vi "Setup.Numeric.Hide.vi"(8 "error in (no error)":errorcluster, 11 "Digital in":refnum<vi>) -> (0 "error out":errorcluster)   [LabVIEW 2015, in "Workspace.Obejct.Radio.lvlib"]
uses:
  Workspace.Obejct.Radio.lvlib
  <vilib>/Utility/miscctls.llb/LVPositionTypeDef.ctl
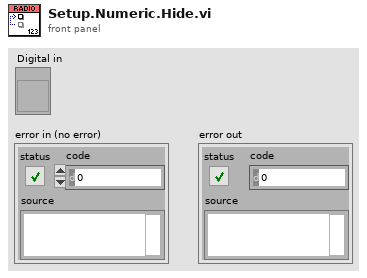
[diagram p1: front panel]
types:
  T1 = typedef "LVPositionTypeDef.ctl" = cluster{"Left":i32, "Top":i32}
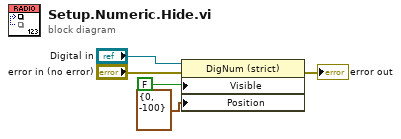
[diagram p0: block diagram]
diagram:
  n1 = property class="DigNum (strict)"(reference="Digital in", error in="error in (no error)", "Visible"=FALSE, "Position"=T1 {"Left"=0, "Top"=-100}) -> (error out=→"error out":errorcluster)  [unwired: 1 out]
